vi "initialize CO1 mainTrig task.vi"(8 "error in (no error)":errorcluster, 11 "NI in":refnum<class "NI.lvclass">) -> (0 "error out":errorcluster, 3 "NI out":refnum<class "NI.lvclass">)   [LabVIEW 2021, in "NI.lvlib" / "NI.lvclass"]
uses:
  NI.lvclass
  NI.lvclass/NI.ctl
  <vilib>/DAQmx/create/channels.llb/DAQmx Create Channel (CO-Pulse Generation-Ticks).vi
  <vilib>/DAQmx/configure/timing.llb/DAQmx Timing (Implicit).vi
  <resource>/objmgr/daqmx.rc
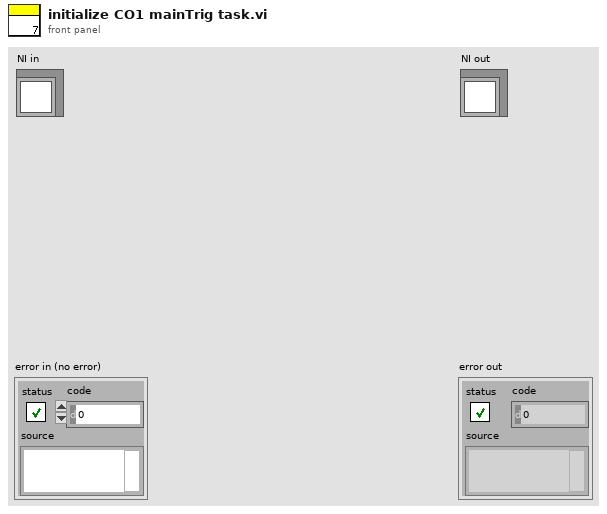
[diagram p1: front panel]
types:
  T1 = typedef "NI.lvlib/NI.lvclass/NI task parameters.ctl" = cluster{"exposure time":dbl, "camera H":dbl, "y line #":dbl, "flyback line #":dbl, "y pixel size":dbl, "z scan #":dbl, "z step size":dbl, "z offset":dbl, "laser all on?":bool, "laser option":bool[]}
  T2 = typedef "NI.lvlib/NI.lvclass/Channel Connection.ctl" = cluster{"Physical Channel":tag, "Terminal":tag, "StartTrigger":tag, "ClockSource":tag}
  T3 = cluster{"fast clock params":cluster{"fast clock rate":dbl, "off time after trigger":dbl, "cam line read time":dbl, "protect ticks #":dbl}, "AO1 laser Connection":T2, "AO2 zy Connection":T2, "AO3 z Connection (deprecated)":T2, "CO1 mainTrig Connection":T2, "CO2 fastClock Connection":T2, "AI phase Connection":T2}
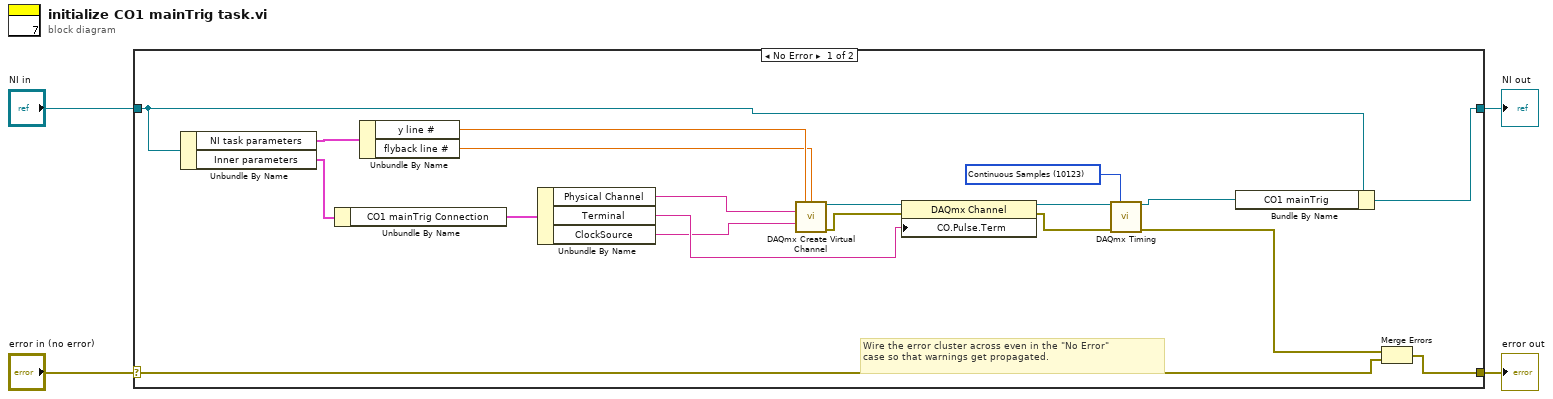
[diagram p0: block diagram]
diagram:
  n1 = case shown="No Error" "error in (no error)" {
    selector: "error in (no error)" -> [w7 w25]
    tunnel: [w6 w25] -> w3
    tunnel: [w9 w24] -> w1
    tunnel: "NI in" -> [w10 w24]
    frame No Error {
      w21 = 10123 items=["Finite Samples"=10178, "Continuous Samples"=10123, "Hardware Timed Single Point"=12522] ("sample mode")
      # "Wire the error cluster across even in the \"No Error\"\ncase so that warnings get propagated."
      n2 = Unbundle By Name(w10) -> ("NI task parameters"=w20:T1, "Inner parameters"=w19:T3)
      n3 = Unbundle By Name(w19) -> ("CO1 mainTrig Connection"=w18:T2)
      n4 = Unbundle By Name(w20) -> ("y line #"=w12:dbl, "flyback line #"=w11:dbl)
      n5 = Unbundle By Name(w18) -> ("Physical Channel"=w17:tag, "Terminal"=w16:tag, "ClockSource"=w15:tag)
      n6 = call-poly <vilib>:"DAQmx Create Virtual Channel.vi"("high ticks"=w12, "low ticks"=w11, "counter"=w17, "source of ticks"=w15) -> ("task out"=w23:refnum<k21>, "error out"=w14:errorcluster)  [unwired: 10 in]
      n7 = property class="DAQmx Channel"(reference=w23, error in=w14, "CO.Pulse.Term"=w16) -> (reference out=w22:refnum<k21>, error out=w13:errorcluster)
      n8 = call-poly <vilib>:"DAQmx Timing.vi"("task/channels in"=w22, "sample mode"=w21, "error in"=w13) -> ("task out"=w8:refnum<k21>, "error out"=w5:errorcluster)  [unwired: 11 in]
      n9 = Bundle By Name(cluster=w10, "CO1 mainTrig"=w8) -> (w9:refnum<class "NI.lvclass">)
      n10 = Merge Errors(w5, w7) -> (w6:errorcluster)
    }
    frame Error {
    }
  }
  "error out" <- w3
  "NI out" <- w1
